vi "Load Rotator.vi"(8 "error in (no error)":errorcluster, 10 "Rotator":dbl, 11 "Acquisition in":refnum<class "Acquisition.lvclass">) -> (0 "error out":errorcluster, 3 "Acquisition out":refnum<class "Acquisition.lvclass">)   [LabVIEW 2018, in "Acquisition.lvclass"]
uses:
  Acquisition.lvclass
  Acquisition.lvclass/Acquisition.ctl
  Channel/Channel.lvclass
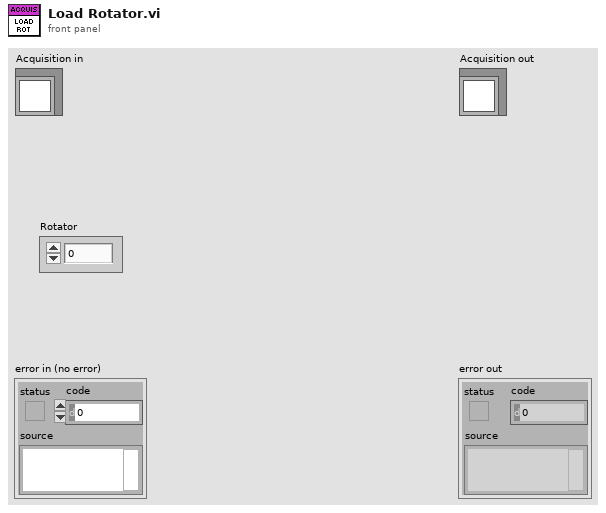
[diagram p1: front panel]
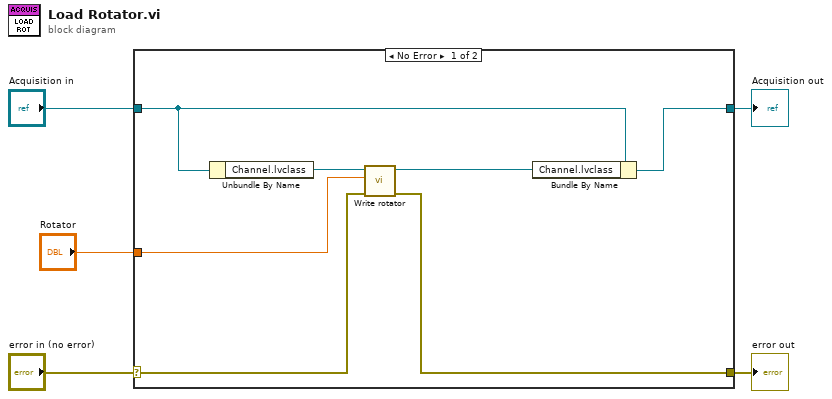
[diagram p0: block diagram]
diagram:
  n1 = case shown="No Error" "error in (no error)" {
    selector: "error in (no error)" -> [w7 w14]
    tunnel: [w6 w14] -> w4
    tunnel: [w11 w13] -> w2
    tunnel: "Acquisition in" -> [w12 w13]
    tunnel: "Rotator" -> [w10 _]
    frame No Error {
      n2 = Unbundle By Name(w12) -> ("Channel.lvclass"=w9:refnum<class "Channel.lvclass">)
      n3 = call-dynamic "Write rotator.vi"("error in (no error)"=w7, "rotator"=w10, "Channel in"=w9) -> ("error out"=w6:errorcluster, "Channel out"=w8:refnum<class "Channel.lvclass">)  [unwired: 7 in]
      n4 = Bundle By Name(cluster=w12, "Channel.lvclass"=w8) -> (w11:refnum<class "Acquisition.lvclass">)
    }
    frame Error {
    }
  }
  "error out" <- w4
  "Acquisition out" <- w2
